vi "Purge_Coils.vi"(3 "Mode":T5, 5 "Traverse line In":T2 {"Row Duration (mins)" format="%#.1f"; "Row No" min=0; "Trace Gas Concentration (%)" min=0.0 format="%#.2f"; "Emission Rate (l/min)" format="%#.2f"; "Tunnel Speed" format="%#.2f"; "Start X" format="%#.2f"; "Start Y" format="%#.2f"; "Start Z" format="%#.2f"; "End X" format="%#.2f"; "End Y" format="%#.2f"; "End Z" format="%#.2f"; "Averaging time (min)" min=0.0 format="%#.1f"}) -> (0 "Error Message":string, 1 "Status":T1, 2 "Traverse line Out":T2 {"Row Duration (mins)" format="%#.1f"; "Row No" min=0; "Trace Gas Concentration (%)" min=0.0 format="%#.2f"; "Emission Rate (l/min)" format="%#.2f"; "Tunnel Speed" format="%#.2f"; "Start X" format="%#.2f"; "Start Y" format="%#.2f"; "Start Z" format="%#.2f"; "End X" format="%#.2f"; "End Y" format="%#.2f"; "End Z" format="%#.2f"; "Averaging time (min)" min=0.0 format="%#.1f"})   [LabVIEW 2010]
uses:
  ADAM Client/Sub VIs/ADAM Controls/Client_Source_Status.ctl
  Gen Trav/Multi_Run_Status.ctl
  Controls/User_Specific_mode.ctl
  Gas desk/Gas desk sub vis/Globals/Timing_Globals_tl.vi
  Gen Trav/Spacing.ctl
  Gen Trav/Traverse_cluster.ctl
  Controls/Multi_run_mode.ctl
panel:
  # "X           Y            Z"
  # "Start"
  # "End"
  # "X           Y            Z"
  # "Start"
  # "End"
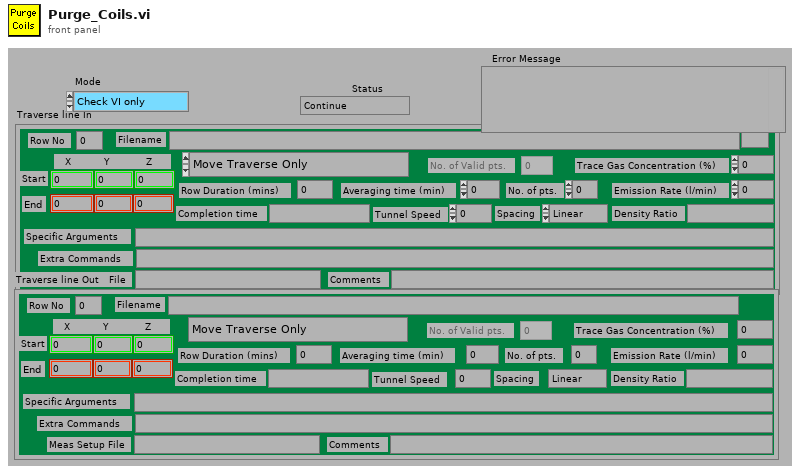
[diagram p1: front panel]
types:
  T1 = typedef "Multi_Run_Status.ctl" = enum16{"Continue", "Jump to Next Point", "Jump to Next Row", "Jump To Fall Back", "Terminate Run"}
  T2 = typedef "Traverse_cluster.ctl" = cluster{"Start X":dbl, "Start Y":dbl, "Start Z":dbl, "End X":dbl, "End Y":dbl, "End Z":dbl, "No. of pts.":i32, "Spacing":T3, "Filename":path, "Tunnel Speed":dbl, "Averaging time (min)":dbl, "Extra Commands":string, "Specific Arguments":string, "Emission Rate (l/min)":dbl, "Trace Gas Concentration (%)":dbl, "Density Ratio":string, "Comments":string, "Row No":i32, "Row Type Selector":T4, "Completion time":string, "Row Duration (mins)":dbl, "No. of Valid pts.":i32, "Meas Setup File":string}
  T3 = typedef "Spacing.ctl" = enum16{"Linear", "Log", "Gauss", "Specified", "N/A"}
  T4 = typedef "Multi_run_mode.ctl" = enum16{"Move Traverse Only", "Set Tunnel Speed Only", "Set Source Only", "Set Measurement Conditions", "Single Measurement", "Vertical Profile", "Lateral Profile", "Longitudinal Profile", "Explore Volume", "Multi-Axis Profile", "Auto Calibrate", "Meas Fast FID Bkgnd", "Check Beam Power", "Scanning Valve Measurement", "Run VI Named:", "Set ADAM Ch", "Wait (minutes)", "Send Message", "Synchronize With:", "Fall Back to this Row", "Turn Off Row Repeating", "Blank Row"}
  T5 = typedef "User_Specific_mode.ctl" = enum16{"Check VI only", "Run VI"}
  T6 = typedef "Client_Source_Status.ctl" = enum16{"Not Using", "Using", "Must Have"}
  T7 = typedef "Status_Cluster.ctl" = cluster{"Status":T1, "Error Type":string, "Error Description":string}
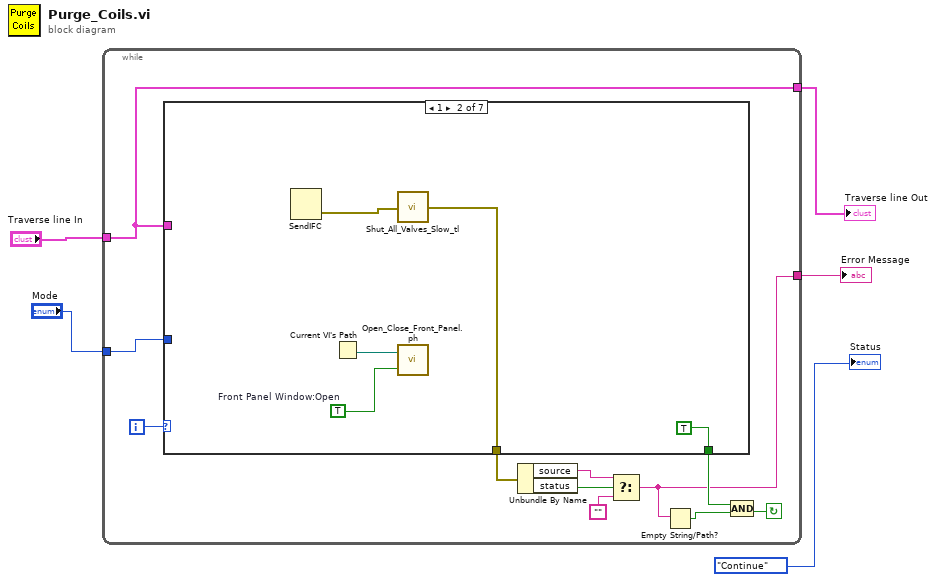
[diagram p0: block diagram]
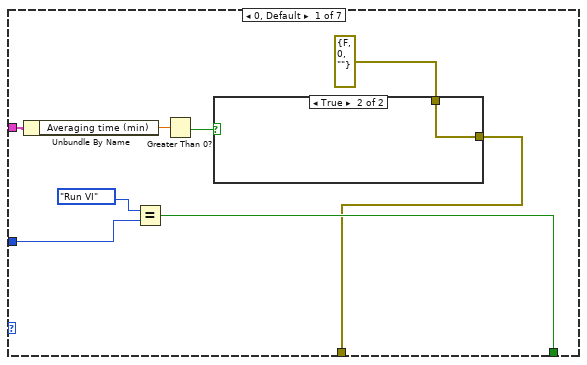
[diagram p2: hidden frame]
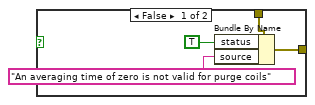
[diagram p3: hidden frame]
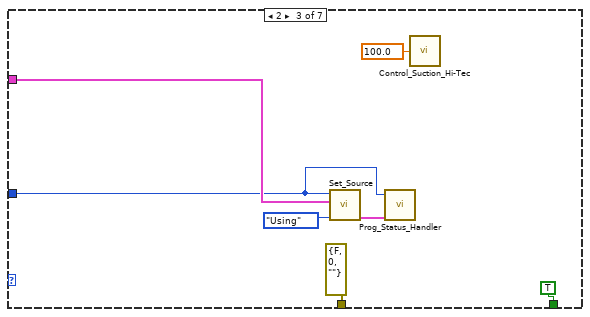
[diagram p4: hidden frame]
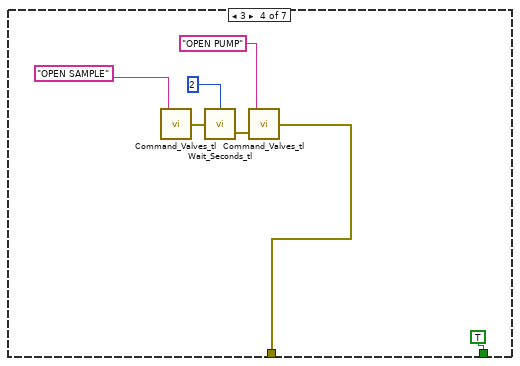
[diagram p5: hidden frame]
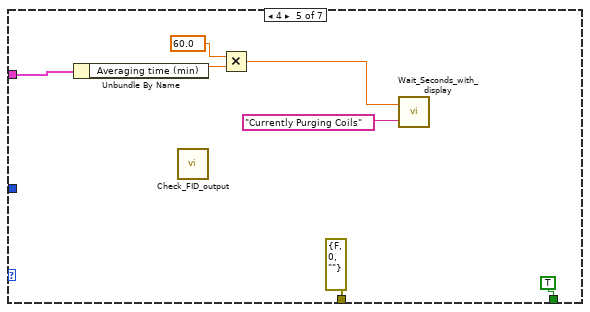
[diagram p6: hidden frame]
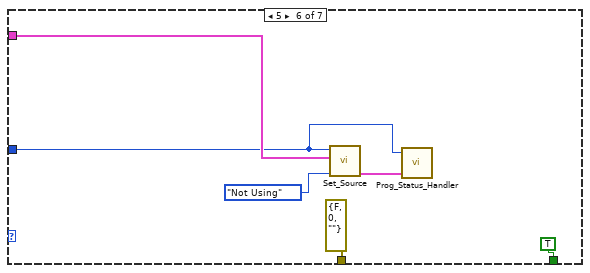
[diagram p7: hidden frame]
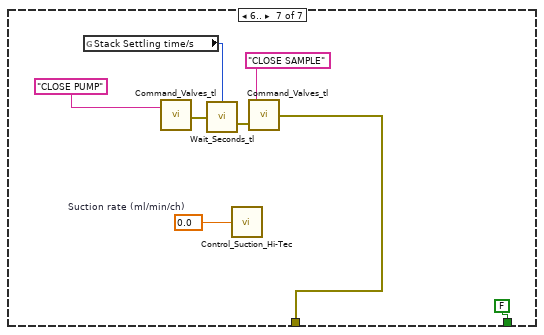
[diagram p8: hidden frame]
diagram:
  n1 = while {
    tunnel: [w6] -> w4
    tunnel: "Mode" -> [w16]
    tunnel: "Traverse line In" -> [w6]
    tunnel: [w7] -> w5
    i -> [w15]
    stop <- w8 continue-if-true
    n2 = case shown="1" w15 {
      tunnel: w6 -> [w21 _ w41 _ w54 w61 _]
      tunnel: w16 -> [w23 _ w35 _ _ w56 _]
      tunnel: [w19 w33 errorcluster {"status"=FALSE, "code"=0, "source"=""} ("error out") w43 errorcluster {"status"=FALSE, "code"=0, "source"=""} ("error out") errorcluster {"status"=FALSE, "code"=0, "source"=""} ("error out") w63] -> w11
      tunnel: [w22 TRUE TRUE TRUE TRUE TRUE FALSE] -> w9
      frame 0, Default {
        n3 = Unbundle By Name(w21) -> ("Averaging time (min)"=w18:dbl)
        n4 = Equal?(x=User_Specific_mode."Run VI" ("Mode"), y=w23) -> (x = y?=w22:bool)
        n5 = Greater Than 0?(x=w18) -> (x > 0?=w17:bool)
        n6 = case shown="True" w17 {
          tunnel: errorcluster {"status"=FALSE, "code"=0, "source"=""} ("error out") -> [w28 w29]
          tunnel: [w27 w29] -> w19
          frame False {
            n7 = Bundle By Name(cluster=w28, "status"=TRUE ("Bundle Element"), "source"="An averaging time of zero is not valid for purge coils" ("Bundle Element")) -> (w27:errorcluster)
          }
          frame True {
          }
        }
      }
      frame 1 {
        w30 = TRUE  # Front Panel Window:Open
        n8 = SendIFC() -> (0:w34:errorcluster)  [unwired: 2 in, 1 out]
        n9 = Current VI's Path() -> (path=w31:path)
        n10 = call "Shut_All_Valves_Slow_tl.vi"("error in"=w34) -> ("error out"=w33:errorcluster)
        n11 = call "Open_Close_Front_Panel.ph.vi"("Front Panel Window:Open"=w30, "VI path"=w31) -> ()  [unwired: 1 in, 1 out]
      }
      frame 2 {
        n12 = call "Set_Source.vi"("Source Status"=Client_Source_Status."Using", "Traverse line"=w41, "Simulate/Run"=w35) -> ("Status Cluster"=w36:T7)  [unwired: 1 in, 5 out]
        n13 = call "Prog_Status_Handler.vi"("Status Cluster"=w36, "Simulate/Run"=w35) -> ()  [unwired: 2 in]
        n14 = call "Control_Suction_Hi-Tec.vi"("Suction rate (ml/min/ch)"=100.0) -> ()  [unwired: 2 out]
      }
      frame 3 {
        n15 = call "Command_Valves_tl.vi"("Command String"="OPEN SAMPLE") -> ("error out"=w46:errorcluster)  [unwired: 1 in]
        n16 = call "Wait_Seconds_tl.vi"("error in"=w46, "Seconds to wait"=u32 2) -> ("error out"=w45:errorcluster)
        n17 = call "Command_Valves_tl.vi"("error in"=w45, "Command String"="OPEN PUMP") -> ("error out"=w43:errorcluster)
      }
      frame 4 {
        n18 = Unbundle By Name(w54) -> ("Averaging time (min)"=w53:dbl)
        n19 = call "Check_FID_output.vi"() -> ()  [unwired: 2 in, 1 out]
        n20 = Multiply(x=60.0, y=w53) -> (x*y=w49:dbl)
        n21 = call "Wait_Seconds_with_display.vi"("Message"="Currently Purging Coils", "Seconds to wait"=w49) -> ()  [unwired: 1 in, 1 out]
      }
      frame 5 {
        n22 = call "Set_Source.vi"("Source Status"=Client_Source_Status."Not Using", "Traverse line"=w61, "Simulate/Run"=w56) -> ("Status Cluster"=w57:T7)  [unwired: 1 in, 5 out]
        n23 = call "Prog_Status_Handler.vi"("Status Cluster"=w57, "Simulate/Run"=w56) -> ()  [unwired: 2 in]
      }
      frame 6.. {
        w64 = 0.0  # Suction rate (ml/min/ch)
        n24 = global read "Timing_Globals_tl.vi" "Stack Settling time/s"() -> (w65:u32)
        n25 = call "Command_Valves_tl.vi"("Command String"="CLOSE PUMP") -> ("error out"=w68:errorcluster)  [unwired: 1 in]
        n26 = call "Wait_Seconds_tl.vi"("error in"=w68, "Seconds to wait"=w65) -> ("error out"=w69:errorcluster)
        n27 = call "Control_Suction_Hi-Tec.vi"("Suction rate (ml/min/ch)"=w64) -> ()  [unwired: 2 out]
        n28 = call "Command_Valves_tl.vi"("error in"=w69, "Command String"="CLOSE SAMPLE") -> ("error out"=w63:errorcluster)
      }
    }
    n29 = Unbundle By Name(w11) -> ("source"=w13:string, "status"=w12:bool)
    n30 = Select(t=w13, s=w12, f="") -> (s? t:f=w7:string)
    n31 = Empty String/Path?(string/path=w7) -> (empty?=w10:bool)
    n32 = Compound Arithmetic op=AND(w9, w10) -> (w8:bool)
  }
  "Error Message" <- w5
  "Traverse line Out" <- w4
  "Status" <- Multi_Run_Status."Continue" ("Status")
